vi "ArrangeValuesByName.vi"(10 "Names":string[](array[string]), 11 "Names/Values in":string[][](array[string])) -> (3 "Names/Values Out":string[][](array[string]))   [LabVIEW 2017]
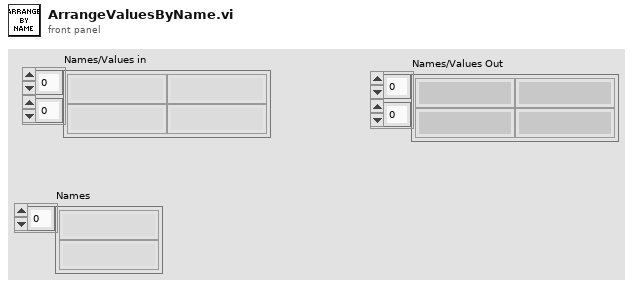
[diagram p1: front panel]
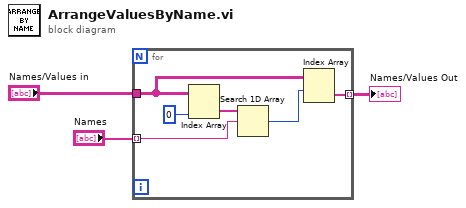
[diagram p0: block diagram]
diagram:
  n1 = for {
    tunnel: "Names" -> [w7] mode=indexing
    tunnel: "Names/Values in" -> [w5]
    tunnel: [w4] -> w1 mode=indexing
    n2 = Index Array(array=w5, index (col)=0 ("disabled index (col)")) -> (element=w8:string[])  [unwired: 1 in]
    n3 = Search 1D Array(1D array=w8, element=w7) -> (index of element=w6:i32)  [unwired: 1 in]
    n4 = Index Array(array=w5, index (row)=w6) -> (element=w4:string[])  [unwired: 1 in]
  }
  "Names/Values Out" <- w1
